vi "Set Direction.vi"(10 "direction":T1, 11 "Transfer Group Configuration in":refnum<class "Transfer Group Configuration.lvclass">) -> (3 "Transfer Group Configuration out":refnum<class "Transfer Group Configuration.lvclass">)   [LabVIEW 2017, in "Data Sharing Framework Core.lvlib" / "Data Sharing Framework Engine.lvlib" / "Transfer Group Configuration.lvclass"]
uses:
  Transfer Group Configuration.lvclass
  Configuration/1.0.0/Public/Controls/DSF Direction.ctl
  Transfer Group Configuration.lvclass/Transfer Group Configuration.ctl
  Configuration/1.0.0/Data Sharing Framework Configuration.lvlib
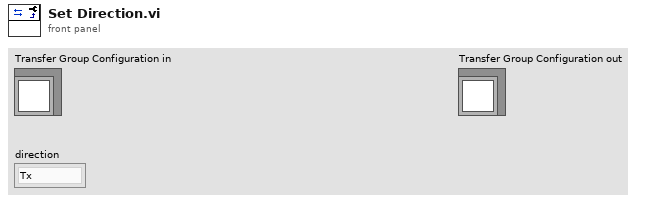
[diagram p1: front panel]
types:
  T1 = typedef "Data Sharing Framework Core.lvlib/Data Sharing Framework Configuration.lvlib/DSF Direction.ctl" = enum8{"Tx", "Rx"}
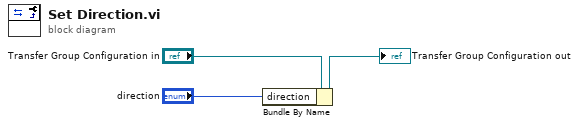
[diagram p0: block diagram]
diagram:
  n1 = Bundle By Name(cluster="Transfer Group Configuration in", "direction"="direction") -> (→"Transfer Group Configuration out":refnum<class "Transfer Group Configuration.lvclass">)
